vi "Test_CheckCommunication.vi"() -> ()   [LabVIEW 2019]
uses:
  ByteRESTLib/CfgLoaders/LoaderBase/ServerParams.ctl
  ByteRESTLib/ByteRESTClass/ByteRESTBase/Auth/Authentication_type.ctl
  ByteRESTLib/CfgLoaders/LoaderConstant/RESTLoaderConstant.lvclass/RESTLoaderConstant.ctl
  ByteRESTLib/ByteRESTClass/ByteRESTBase/RESTBase.lvclass
  ByteRESTLib/CfgLoaders/LoaderConstant/RESTLoaderConstant.lvclass
  C:/Users/AlessandroPerla/Desktop/prj_local/BytelabsLibraryDev/ByteREST/ByteRESTLib/CfgLoaders/LoaderBase/RESTLoaderBase.lvclass
  ByteRESTLib/CfgLoaders/LoaderBase/RESTLoaderBase.lvclass
panel:
  out "Passed":bool
  out "error out":errorcluster
  out "Body":string
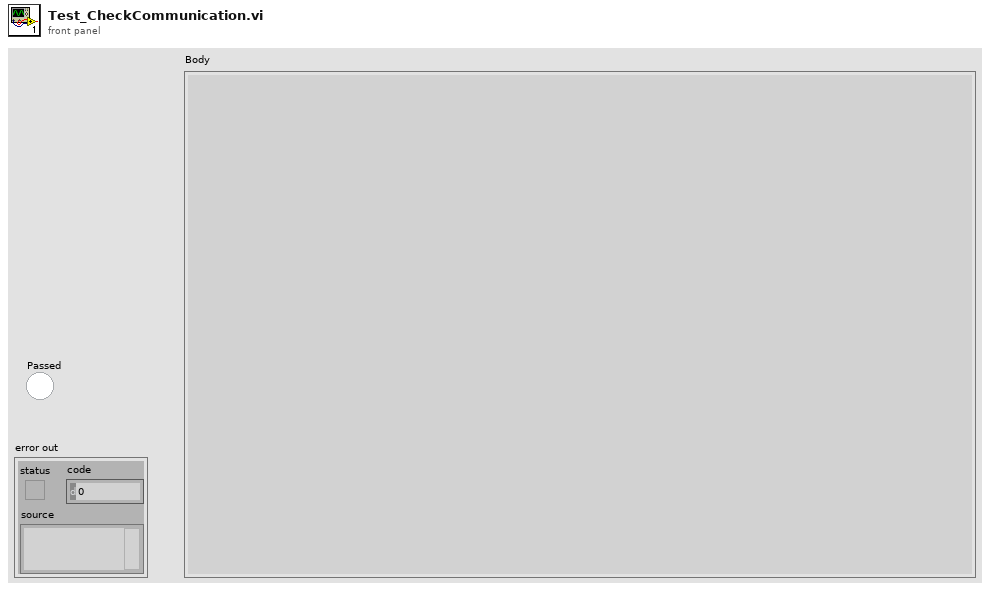
[diagram p1: front panel]
types:
  T1 = typedef "ByteREST.lvlib/RESTLoaderBase.lvclass/ServerParams.ctl" = cluster{"API Root":string, "verify server":bool, "Version (no version)":string, "Port (protocol specific)":u16, "Base URL":string, "Auth type":T2, "Auth string":string, "timeout (10000)":i32, "Token preamble (Token)":string, "Token empty preamble (False)":bool, "Token header key (Authorization)":string}
  T2 = typedef "ByteREST.lvlib/RESTBase.lvclass/Authentication_type.ctl" = enum16{"Token"}
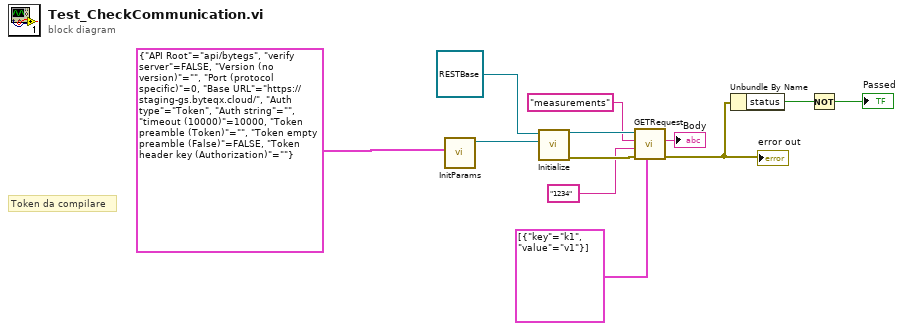
[diagram p0: block diagram]
diagram:
  # "Token da compilare"
  n1 = call "InitParams.vi"("Cluster"=T1 {"API Root"="api/bytegs", "verify server"=FALSE, "Version (no version)"="", "Port (protocol specific)"=0, "Base URL"="https://staging-gs.byteqx.cloud/", "Auth type"=enum."Token", "Auth string"="", "timeout (10000)"=10000, "Token preamble (Token)"="", "Token empty preamble (False)"=FALSE, "Token header key (Authorization)"=""}) -> ("RESTLoaderConstant out"=w11:refnum<class "RESTLoaderConstant.lvclass">)  [unwired: 10 in]
  n2 = call-dynamic "Initialize.vi"("RESTLoader"=w11, "REST in"=refnum<class "RESTBase.lvclass"> refnum) -> ("error out"=w7:errorcluster, "REST out"=w9:refnum<class "RESTBase.lvclass">)  [unwired: 8 in]
  n3 = call-dynamic "GETRequest.vi"("Query parameters"=cluster{"key":string, "value":string}[] [{"key"="k1", "value"="v1"}], "error in (no error)"=w7, "Parameter"="1234", "Request"="measurements", "ByteRESTBase in"=w9) -> ("error out"=w5:errorcluster, "Body"=→"Body":string)  [unwired: 3 in, 2 out]
  "error out" <- w5
  n4 = Unbundle By Name(w5) -> ("status"=w4:bool)
  n5 = Not(x=w4) -> (.not. x?=→"Passed":bool)
